vi "Write.Encrypted.7zPayload.vi"(8 "error in (no error)":errorcluster, 9 "Password":string="pw", 11 "File Path":path) -> (0 "error out":errorcluster, 3 "7z Path Out":path)   [LabVIEW 2020, in "PixPack.lvlib"]
uses:
  PixPack.lvlib
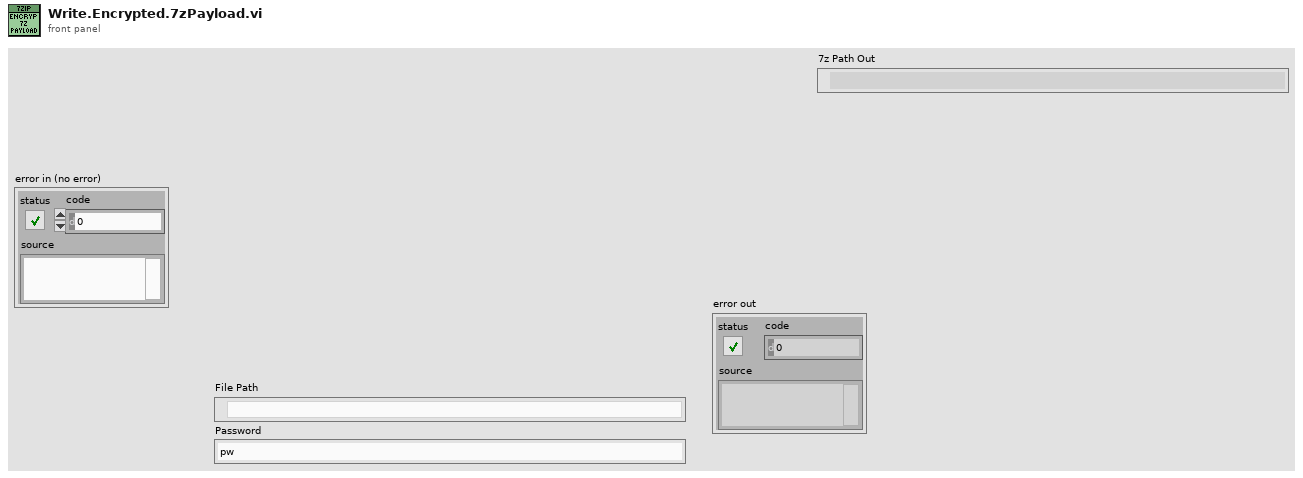
[diagram p1: front panel]
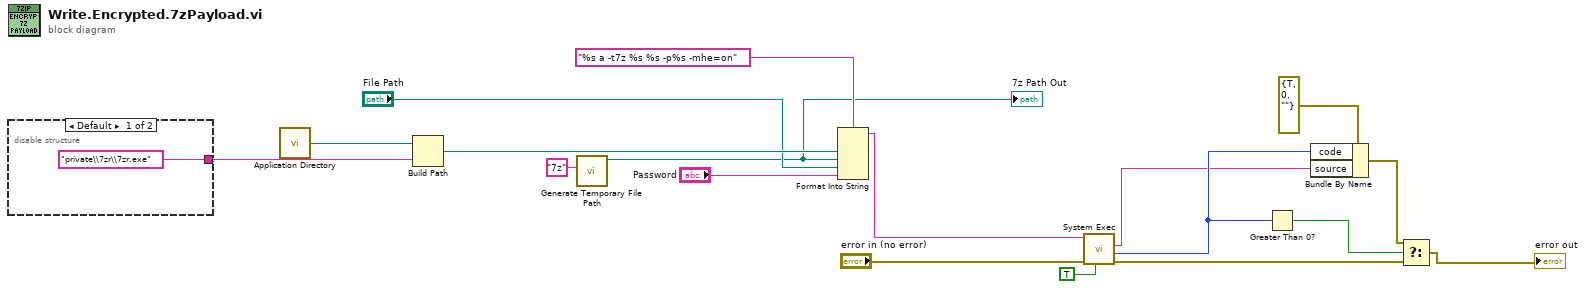
[diagram p0: block diagram]
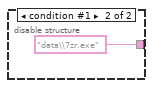
[diagram p2: hidden frame]
diagram:
  n1 = disable-structure shown="Default" {
    disable-tunnel: ["private\\7zr\\7zr.exe" "data\\7zr.exe"] -> w17
    frame condition #0 (active) {
    }
    frame condition #1 {
    }
  }
  n2 = call <vilib>:"Application Directory.vi"() -> ("Application Directory"=w16:path)
  n3 = Build Path(base path=w16, name or relative path=w17) -> (appended path=w10:path)
  n4 = call <vilib>:"Generate Temporary File Path.vi"("Temporary File Extension (tmp)"="7z") -> ("Unique Temporary File Path"=w8:path)  [unwired: 9 in, 1 out]
  "7z Path Out" <- w8
  n5 = Format Into String(format string="%s a -t7z %s %s -p%s -mhe=on", w10, w8, "File Path", "Password") -> (resulting string=w13:string)  [unwired: 2 in, 1 out]
  n6 = call <vilib>:"System Exec.vi"("run minimized? (F)"=TRUE, "error in (no error)"="error in (no error)", "command line"=w13) -> ("error out"=w4:errorcluster, "return code"=w3:i32, "standard error"=w2:string)  [unwired: 5 in, 1 out]
  n7 = Greater Than 0?(x=w3) -> (x > 0?=w7:bool)
  n8 = Bundle By Name(cluster=errorcluster {"status"=TRUE, "code"=0, "source"=""} ("error out"), "code"=w3, "source"=w2) -> (w5:errorcluster)
  n9 = Select(t=w5, s=w7, f=w4) -> (s? t:f=→"error out":errorcluster)
